vi "Write Network Master.vi"(8 "error in":errorcluster, 10 "network master":refnum<class "Network Master.lvclass">, 11 "Modbus master in":refnum<class "Modbus Master.lvclass">) -> (0 "error out":errorcluster, 3 "Modbus master out":refnum<class "Modbus Master.lvclass">)   [LabVIEW 2015, in "Modbus Library.lvlib" / "Modbus Master.lvclass"]
doc: "This VI is an accessor for the <B>network master</B> stored in the Modbus master instance. This accessor can be used as a property node. This network master is used by the Modbus instance to communicate on the physical bus."
uses:
  Modbus Master.lvclass
  Network Protocol/Network Master/Network Master.lvclass
  Modbus Master.lvclass/Modbus Master.ctl
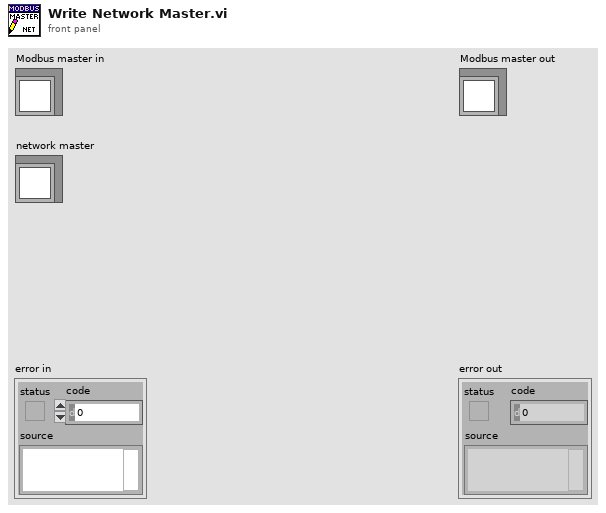
[diagram p1: front panel]
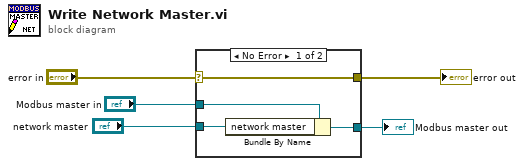
[diagram p0: block diagram]
diagram:
  n1 = case shown="No Error" "error in" {
    selector: "error in" -> [w9 w10]
    tunnel: [w9 w10] -> w4
    tunnel: [w7 w11] -> w2
    tunnel: "Modbus master in" -> [w8 w11]
    tunnel: "network master" -> [w6 _]
    frame No Error {
      n2 = Bundle By Name(cluster=w8, "network master"=w6) -> (w7:refnum<class "Modbus Master.lvclass">)
    }
    frame Error {
    }
  }
  "error out" <- w4
  "Modbus master out" <- w2
